vi "FTW-JSON-CompareEquality.vi"(0 "JSON Object":refnum<data-value>, 5 "JSON Object to Compare":refnum<data-value>, 11 "error in":errorcluster) -> (4 "Equal?":bool, 15 "error out":errorcluster)   [LabVIEW 2014]
uses:
  core/FTW-JSON-Core-Structure.ctl
  error/FTW-ERR-ThrowGenericError.vi
  error/FTW-ERR-ThrowError.vi
  error/FTW-ERR-NoErrorConstant.vi
  error/FTW-ERR-CallChain.vi
  string/FTW-STR-ReplaceWhitespace.vi
panel:
  # "Inputs"
  # "Outputs"
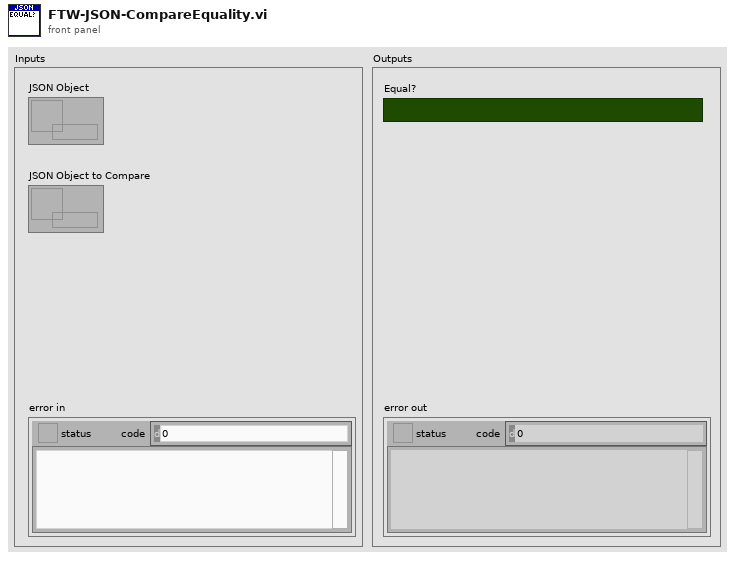
[diagram p1: front panel]
types:
  T1 = typedef "FTW-JSON-Core-Structure.ctl" = cluster{"JSON Object":i64, "Encoding Flags":i64, "Decoding Flags":i64}
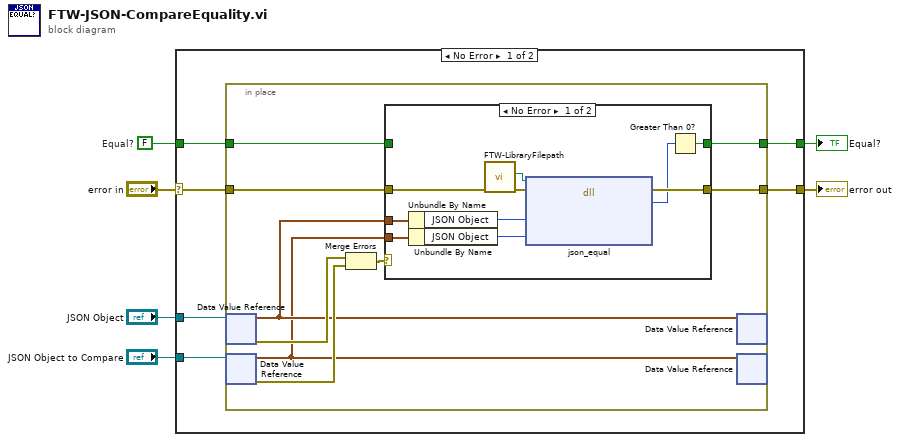
[diagram p0: block diagram]
diagram:
  w1 = FALSE  # Equal?
  n1 = case shown="No Error" "error in" {
    selector: "error in" -> [w12 w35]
    tunnel: [w11 w35] -> w6
    tunnel: "JSON Object" -> [w9 _]
    tunnel: [w10 w34] -> w3
    tunnel: "JSON Object to Compare" -> [w8 _]
    tunnel: w1 -> [w7 w34]
    frame No Error {
      n2 = in-place {
        in-place-border: w12 -> [w21]
        in-place-border: [w20] -> w11
        in-place-border: [w19] -> w10
        in-place-border: w7 -> [w15]
        n3 = in-place-dvr #1(w9) -> (w14:T1, w18:errorcluster)
        n4 = in-place-dvr #2(w8) -> (w13:T1, w17:errorcluster)
        n5 = Merge Errors(w18, w17) -> (w16:errorcluster)
        n6 = case shown="No Error" w16 {
          tunnel: w21 -> [w31 w33]
          tunnel: [w30 w33] -> w20
          tunnel: [w26 w32] -> w19
          tunnel: w15 -> [_ w32]
          tunnel: w14 -> [w23 _]
          tunnel: w13 -> [w22 _]
          frame No Error {
            n7 = Unbundle By Name(w23) -> ("JSON Object"=w25:i64)
            n8 = Unbundle By Name(w22) -> ("JSON Object"=w24:i64)
            n9 = call "FTW-LibraryFilepath.vi"("error in"=w31) -> ("error out"=w28:errorcluster, "Library Filepath"=w27:path)  [unwired: 8 in, 1 out]
            n10 = dll-call lib="?" fn="json_equal"(path in=w27, error in=w28, "JSON Object Pointer 1"=w25, "JSON Object Pointer 2"=w24) -> (error out=w30:errorcluster, "Are Objects Equal?"=w29:u8)  [unwired: 3 in, 1 out]
            n11 = Greater Than 0?(x=w29) -> (x > 0?=w26:bool)
          }
          frame Error {
          }
        }
        n12 = in-place-dvr #1(w14) -> ()  [unwired: 2 out]
        n13 = in-place-dvr #2(w13) -> ()  [unwired: 2 out]
      }
    }
    frame Error {
    }
  }
  "error out" <- w6
  "Equal?" <- w3
